vi "Get Address from Cluster.vi"(4 "Class Attributes":T1) -> (1 "Address":string)   [LabVIEW 2015]
uses:
  Instrument Drivers/Controls/Class Attributes Cluster.ctl
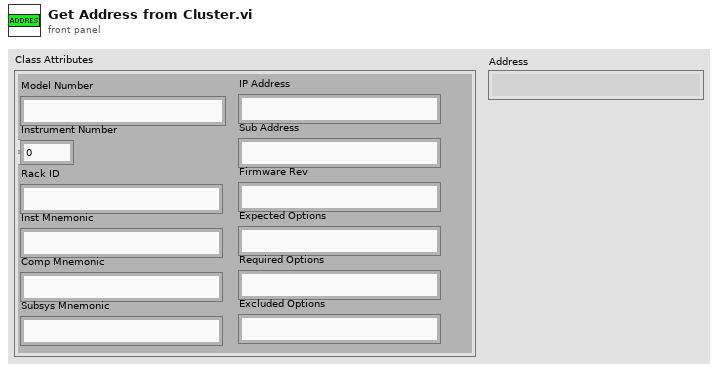
[diagram p1: front panel]
types:
  T1 = typedef "Class Attributes Cluster.ctl" = cluster{"Model Number":string, "Instrument Number":u8, "Rack ID":string, "Inst Mnemonic":string, "Comp Mnemonic":string, "Subsys Mnemonic":string, "IP Address":string, "Sub Address":string, "Firmware Rev":string, "Expected Options":string, "Required Options":string, "Excluded Options":string}
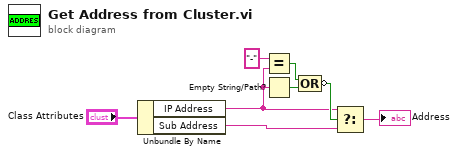
[diagram p0: block diagram]
diagram:
  n1 = Unbundle By Name("Class Attributes") -> ("IP Address"=w1:string, "Sub Address"=w2:string)
  n2 = Equal?(x="-", y=w1) -> (x = y?=w6:bool)
  n3 = Empty String/Path?(string/path=w1) -> (empty?=w5:bool)
  n4 = Compound Arithmetic op=OR(w6, w5) -> (invert w7:bool)
  n5 = Select(t=w1, s=w7, f=w2) -> (s? t:f=→"Address":string)
